vi "FTW-Actor-Destroy.vi"(0 "FTW Actor":refnum<class "FTW-Actor.lvclass">, 11 "error in":errorcluster) -> (15 "error out":errorcluster)   [LabVIEW 2013, in "FTW-Actor.lvclass"]
uses:
  FTW-Actor.lvclass
  FTW-Actor.lvclass/FTW-Actor.ctl
  Sequencer/FTW-Sequencer.lvclass
  Context/Messaging/Broker/FTW-Actor-Broker.lvclass
panel:
  # "Inputs"
  # "Outputs"
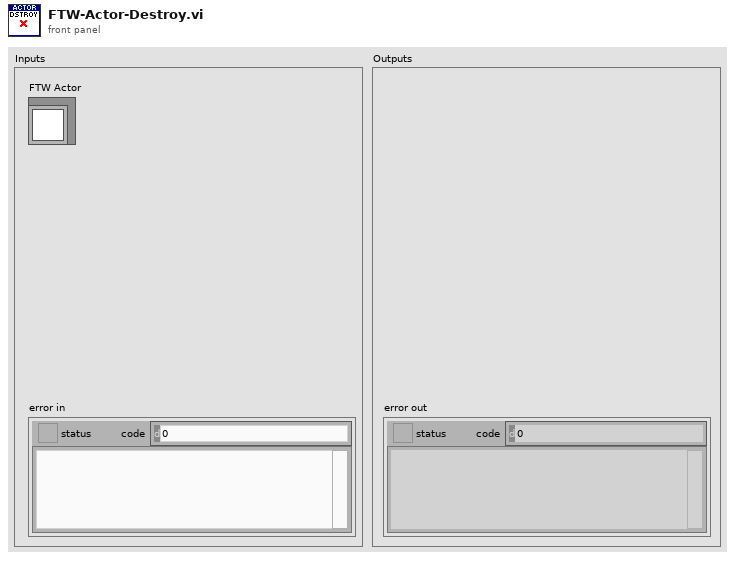
[diagram p1: front panel]
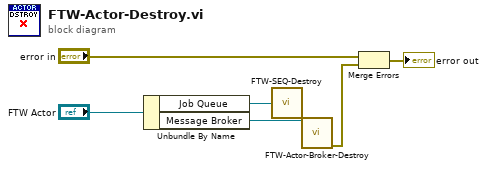
[diagram p0: block diagram]
diagram:
  n1 = Unbundle By Name("FTW Actor") -> ("Job Queue"=w3:refnum<class "FTW-Sequencer.lvclass">, "Message Broker"=w2:refnum<class "FTW-Actor-Broker.lvclass">)
  n2 = call "FTW-SEQ-Destroy.vi"("Sequencer"=w3) -> ()  [unwired: 1 in]
  n3 = call "FTW-Actor-Broker-Destroy.vi"("FTW Message Broker"=w2) -> ("error out"=w1:errorcluster)  [unwired: 14 in]
  n4 = Merge Errors("error in", w1) -> (→"error out":errorcluster)
